vi "Camera.v11.vi"() -> ()   [LabVIEW 2015]
uses:
  Camera Properties.ctl
  Microscope Settings.ctl
  CameraState.ctl
  CameraControlTypeDef.ctl
  ModeEnum.ctl
  Stack Track.ctl
  Stack_State.ctl
  <vilib>/DAQmx/write.llb/DAQmx Write (Digital 1D Wfm NChan NSamp).vi
  <vilib>/DAQmx/write.llb/DAQmx Write (Analog 1D Wfm NChan NSamp).vi
  <vilib>/DAQmx/create/channels.llb/DAQmx Create Channel (AO-Voltage-Basic).vi
  <vilib>/DAQmx/create/channels.llb/DAQmx Create Channel (DO-Digital Output).vi
  <vilib>/Waveform/DWDTOps.llb/DWDT Append Digital Samples.vi
  <vilib>/Waveform/WDTOps.llb/WDT Append Waveforms DBL.vi
  <vilib>/Waveform/WDTOps.llb/WDT Number of Waveform Samples DBL.vi
  <vilib>/DAQmx/configure/timing.llb/DAQmx Timing (Sample Clock).vi
  <vilib>/Waveform/DWDTOps.llb/DWDT Uncompress Digital.vi
  <vilib>/DAQmx/miscellaneous.llb/DAQmx Fill In Error Info.vi
  <vilib>/vision/NI_Vision_Development_Module.lvlib
panel:
  in  "Tab Control":enum32{"Camera Settings", "Recording"}(tab)
  in  "Scans":dbl=1.0 min=0.0 max=10.0 step=0.05
  in  "?":bool
  in  "Microscope Settings":T1={"Mode"=enum."XY", "Slit"={"Scanning Mode"=12.0, "Slit Width /%"=5.0}, "Colour"=[{"Laser"=enum."561", "Filter"=4}], "Exposure/ms"=40.0, "Piezo Position /um"=0.0, "ROI"={"X"={"Start"=0.0, "Step"=1.0, "Range"=2048.0}, "Y"={"Start"=0.0, "Step"=1.0, "Range"=2048.0}, "Z "={"Start"=0.0, "Step"=1.0, "Range"=100.0}}, "Samples per millisecond"=100.0, "Relax/ms"=10.0, "Readout Direction"=2.0, "Trigger Source"=2.0, "Camera Delay /ms"=11.0, "Under Scan"=5.0} {"Under Scan" min=0.0 max=10.0 step=0.05; "ROI"."X"."Range" min=0.0 max=10.0 step=0.05; "ROI"."X"."Step" min=0.0 max=10.0 step=0.05; "ROI"."X"."Start" min=0.0 max=10.0 step=0.05; "ROI"."Y"."Range" min=0.0 max=10.0 step=0.05; "ROI"."Y"."Step" min=0.0 max=10.0 step=0.05; "ROI"."Y"."Start" min=0.0 max=10.0 step=0.05; "ROI"."Z"."Range" min=0.0 max=10.0 step=0.05; "ROI"."Z"."Step" min=0.0 max=10.0 step=0.05; "ROI"."Z"."Start" min=0.0 max=10.0 step=0.05; "Colour"."Filter" items=["Empty"=1, ""=2, ""=3, "561"=4, ""=5, "488"=6]; "Camera Delay /ms" min=0.0 max=10.0 step=0.05; "Trigger Source" items=["Internal"=1.0, "External"=2.0]; "Readout Direction" items=["Forward"=1.0, "Backward"=2.0]; "Slit"."Scanning Mode" items=["Full Frame"=1.0, "Slit Scanning"=12.0]; "Piezo Position /um" min=0.0 max=10.0 step=0.05}
  in  "Scan":bool
  in  "Scan Continuously":bool
  out "error IO":errorcluster
  in  "Advanced DCAM Controls":i32(listbox) caption="Multicolumn Listbox"
  in  "Properties":T2=4211904 items=["SENSOR MODE"=4212128, "CCD MODE"=4212384, "READOUT MODE"=4211872, "ACTIVE VIEW INDEX"=4343136, "BITS PER CHANNEL"=4342976, "IMAGE PIXEL TYPE"=4343296, "BINNING"=4215968, "EXPOSURE TIME"=2049184, "CONTRAST GAIN"=3163312, "CONTRAST OFFSET"=3163328, "LIGHT MODE"=2114720, "SENSITIVITY"=2114992, "PHOTON IMAGING MODE"=2115200, "HIGH DYNAMIC RANGE MODE"=3163360, "WHITE BALANCE"=3163568, "TEMPERATURE"=2115232, "TEMPERATURE TARGET"=2115264, "SENSOR COOLER FAN"=2115296, "LINEBUNDLE HEIGHT"=4212192, "MECHANICAL SHUTTER"=2115488, "BACK FOCUS POSITION"=8422304, "TRIGGER CONNECTOR"=1066432, "TRIGGER SOURCE"=1066144, "OUTPUT TRIGGER SOURCE"=1852576, "TRIGGER GLOBAL EXPOSURE"=2049680, "FIRST TRIGGER BEHAVIOR"=2049696, "CHANNEL SYNC"=1852352, "READOUT DIRECTION"=4211904, "PRE HSYNC COUNT"=1852704, "INTERNAL LINE SPEED"=4191408, "INTERNAL LINE INVERVAL"=4191424]
  out "appended path":path
  in  "Frames":i32
  in  "Imaging Folder":path=path "C:/_DATA/test/a.tif"
  in  "Multicolumn Listbox":i32(listbox)
  out "Image":T3(plugin-control)
  out "Histogram":T4(graph)
  in  "stop":bool
  in  "Record":bool
  in  "Signals Debugger":bool
  in  "Calibration":bool
  in  "MultiD Scan":bool
  in  "Stage Controller":bool
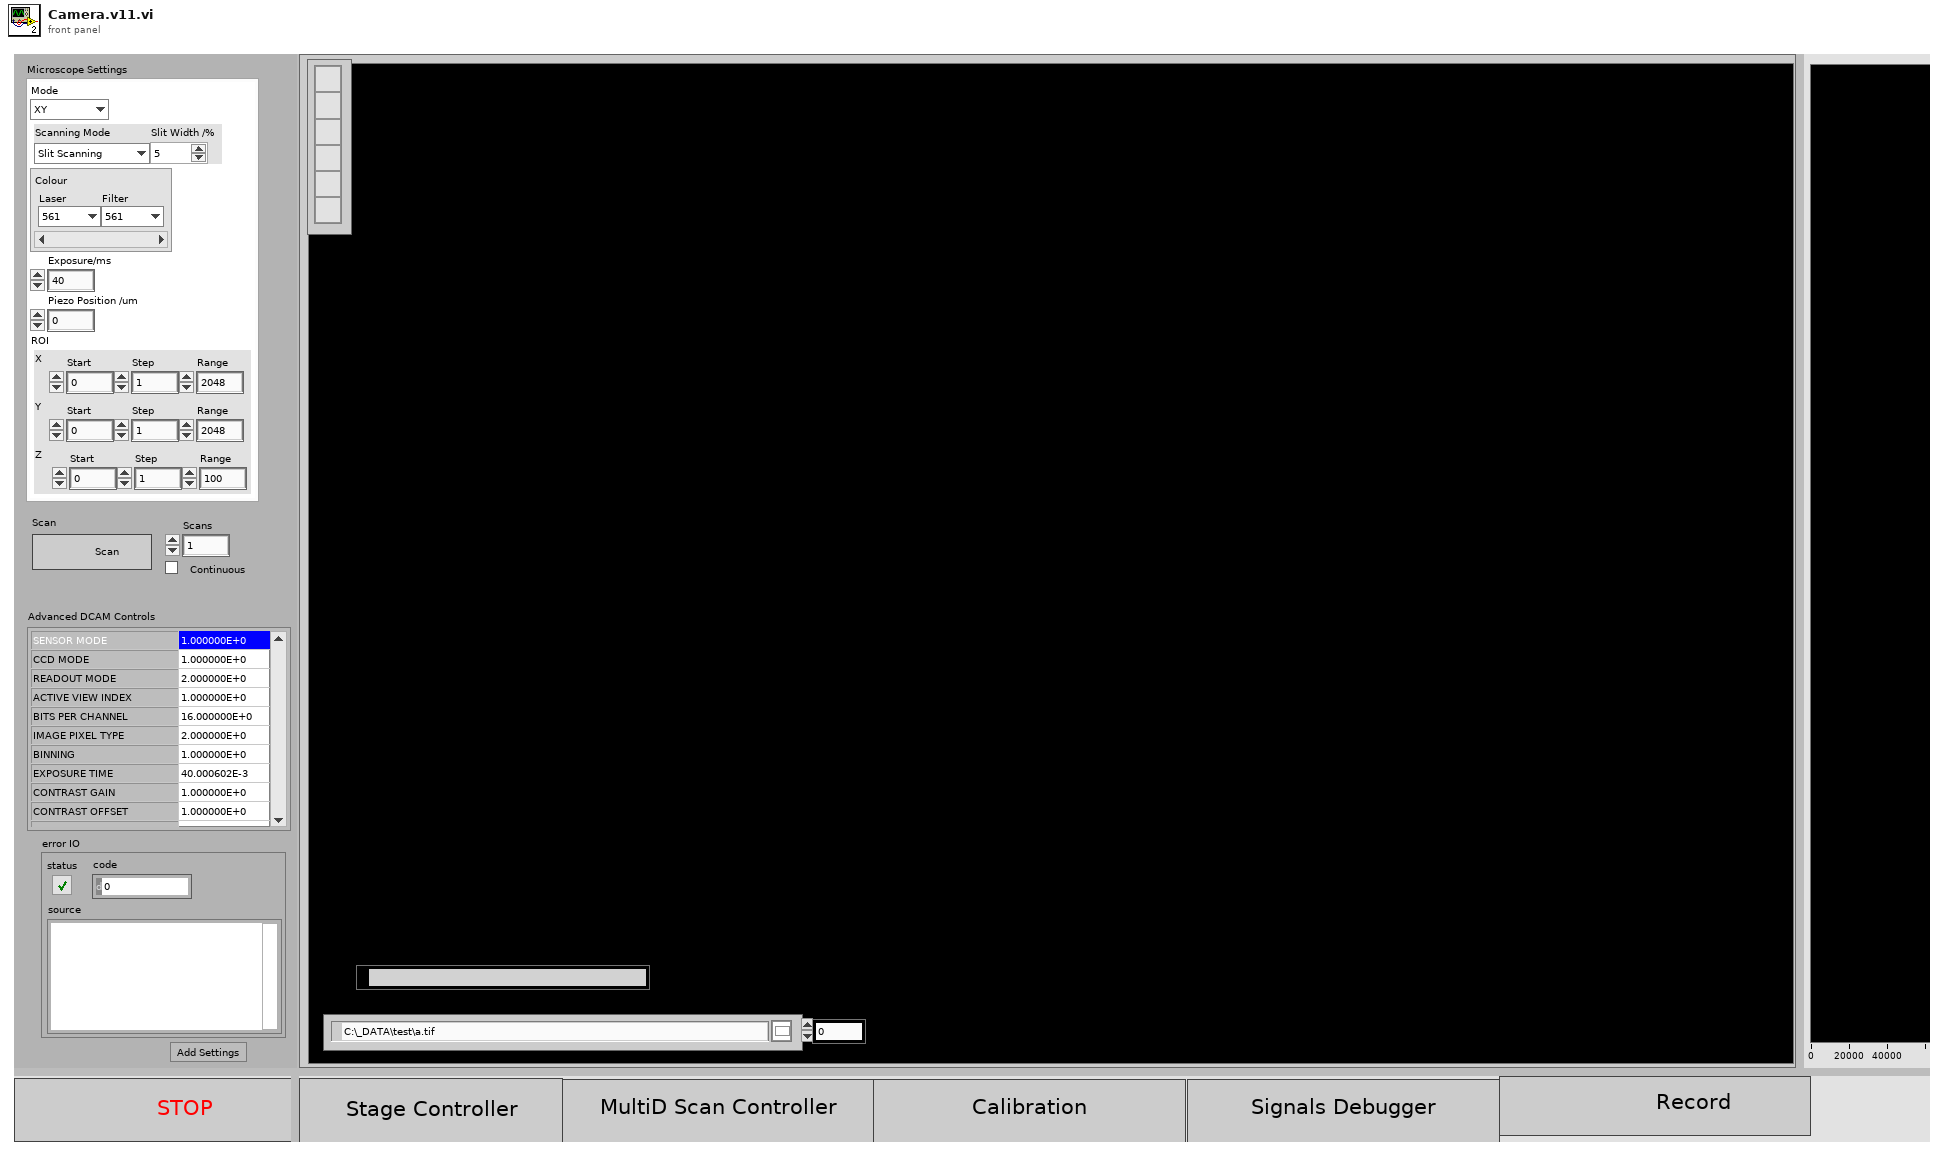
[diagram p1: front panel]
types:
  T1 = typedef "Microscope Settings.ctl" = cluster{"Mode":enum16{"X", "XY", "XYZ", "XYZT", "XYZC"}, "Slit":cluster{"Scanning Mode":dbl, "Slit Width /%":dbl}, "Colour":cluster{"Laser":enum16{"Brightfield", "445", "488", "561", "647"}, "Filter":u16}[], "Exposure/ms":dbl, "Piezo Position /um":dbl, "ROI":cluster{"X":cluster{"Start":dbl, "Step":dbl, "Range":dbl}, "Y":cluster{"Start":dbl, "Step":dbl, "Range":dbl}, "Z ":cluster{"Start":dbl, "Step":dbl, "Range":dbl}}, "Samples per millisecond":dbl, "Relax/ms":dbl, "Readout Direction":dbl, "Trigger Source":dbl, "Camera Delay /ms":dbl, "Under Scan":dbl}
  T2 = typedef "Camera Properties.ctl" = u32
  T3 = typedef "IMAQ Image.ctl" = refnum<image>
  T4 = cluster{"Starting Value":sgl, "Incremental Value":sgl, "Histogram":u32[]}
  T5 = cluster{"height":u32, "width":u32, "datatype":u32}
  T6 = typedef "CameraState.ctl" = enum16{"init", "active", "deinit"}
  T7 = typedef "ModeEnum.ctl" = enum16{"Idle", "generateWaves", "runWaves", "stop"}
  T8 = typedef "CameraControlTypeDef.ctl" = enum16{"Idle", "IntervalLineInt", "Ram Record", "HardDisk Record", "Disengage Update", "Update", "ROI", "Binning", "Scan Mode", "Trigger Mode", "Readout Mode", "Readout Direction", "Preview", "ROIWindow", "Trigger Source"}
  T9 = cluster{"Mode":u32, "Polarity":u32, "Times":u32, "Delay":dbl}
  T10 = typedef "Stack_State.ctl" = cluster{"State":T11, "Stack Number":i32, "Image":u16[][], "Stacks":i32}
  T11 = typedef "Stack Track.ctl" = enum16{"Idle", "Display", "Start Sequence", "Read Disk", "STOP", "Collecting", "End", "Save Image"}
  T12 = enum32{"Invalid", "Standard", "Closed", "Hidden", "Minimized", "Maximized"}
  T13 = typedef "Image Type" = u32
  T14 = cluster{"Analogue Out":waveform(dbl)[], "Digital Out":digitalwaveform[]}
  T15 = cluster{"State":T11, "Timeout":i32, "Data 16":u16[][], "Timeout":i32}
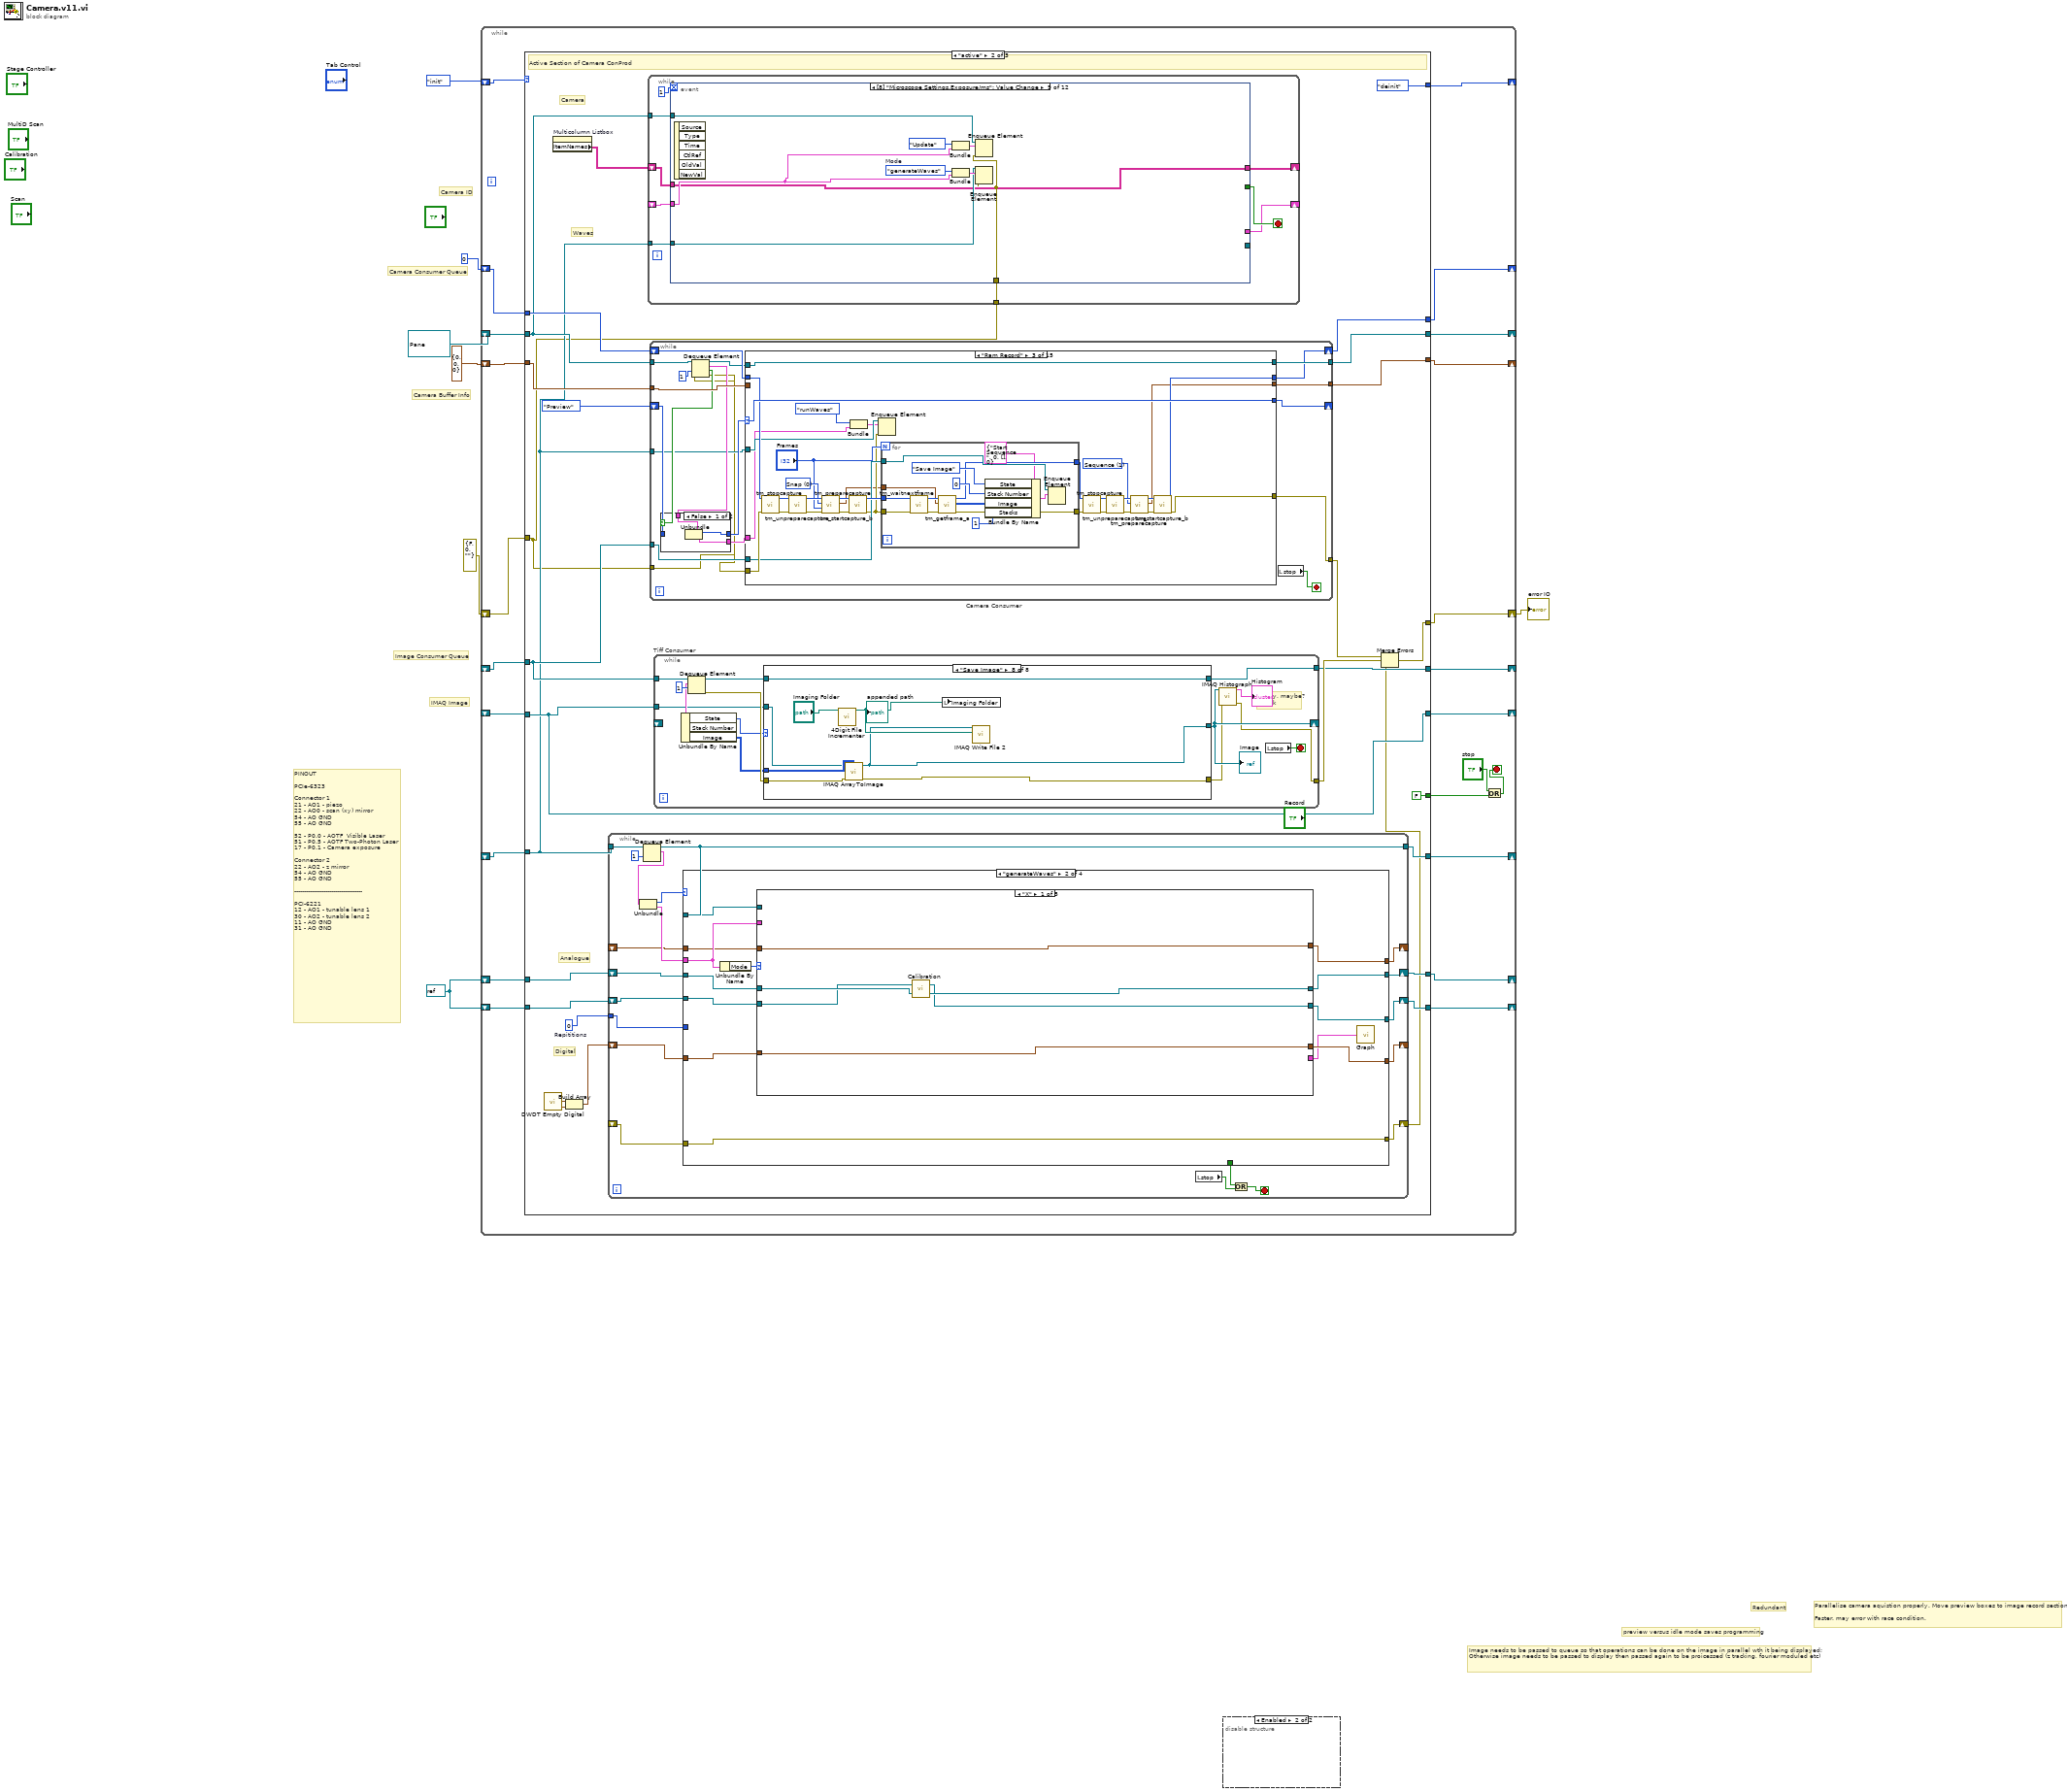
[diagram p0: block diagram]
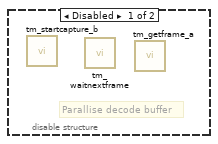
[diagram p2: hidden frame]
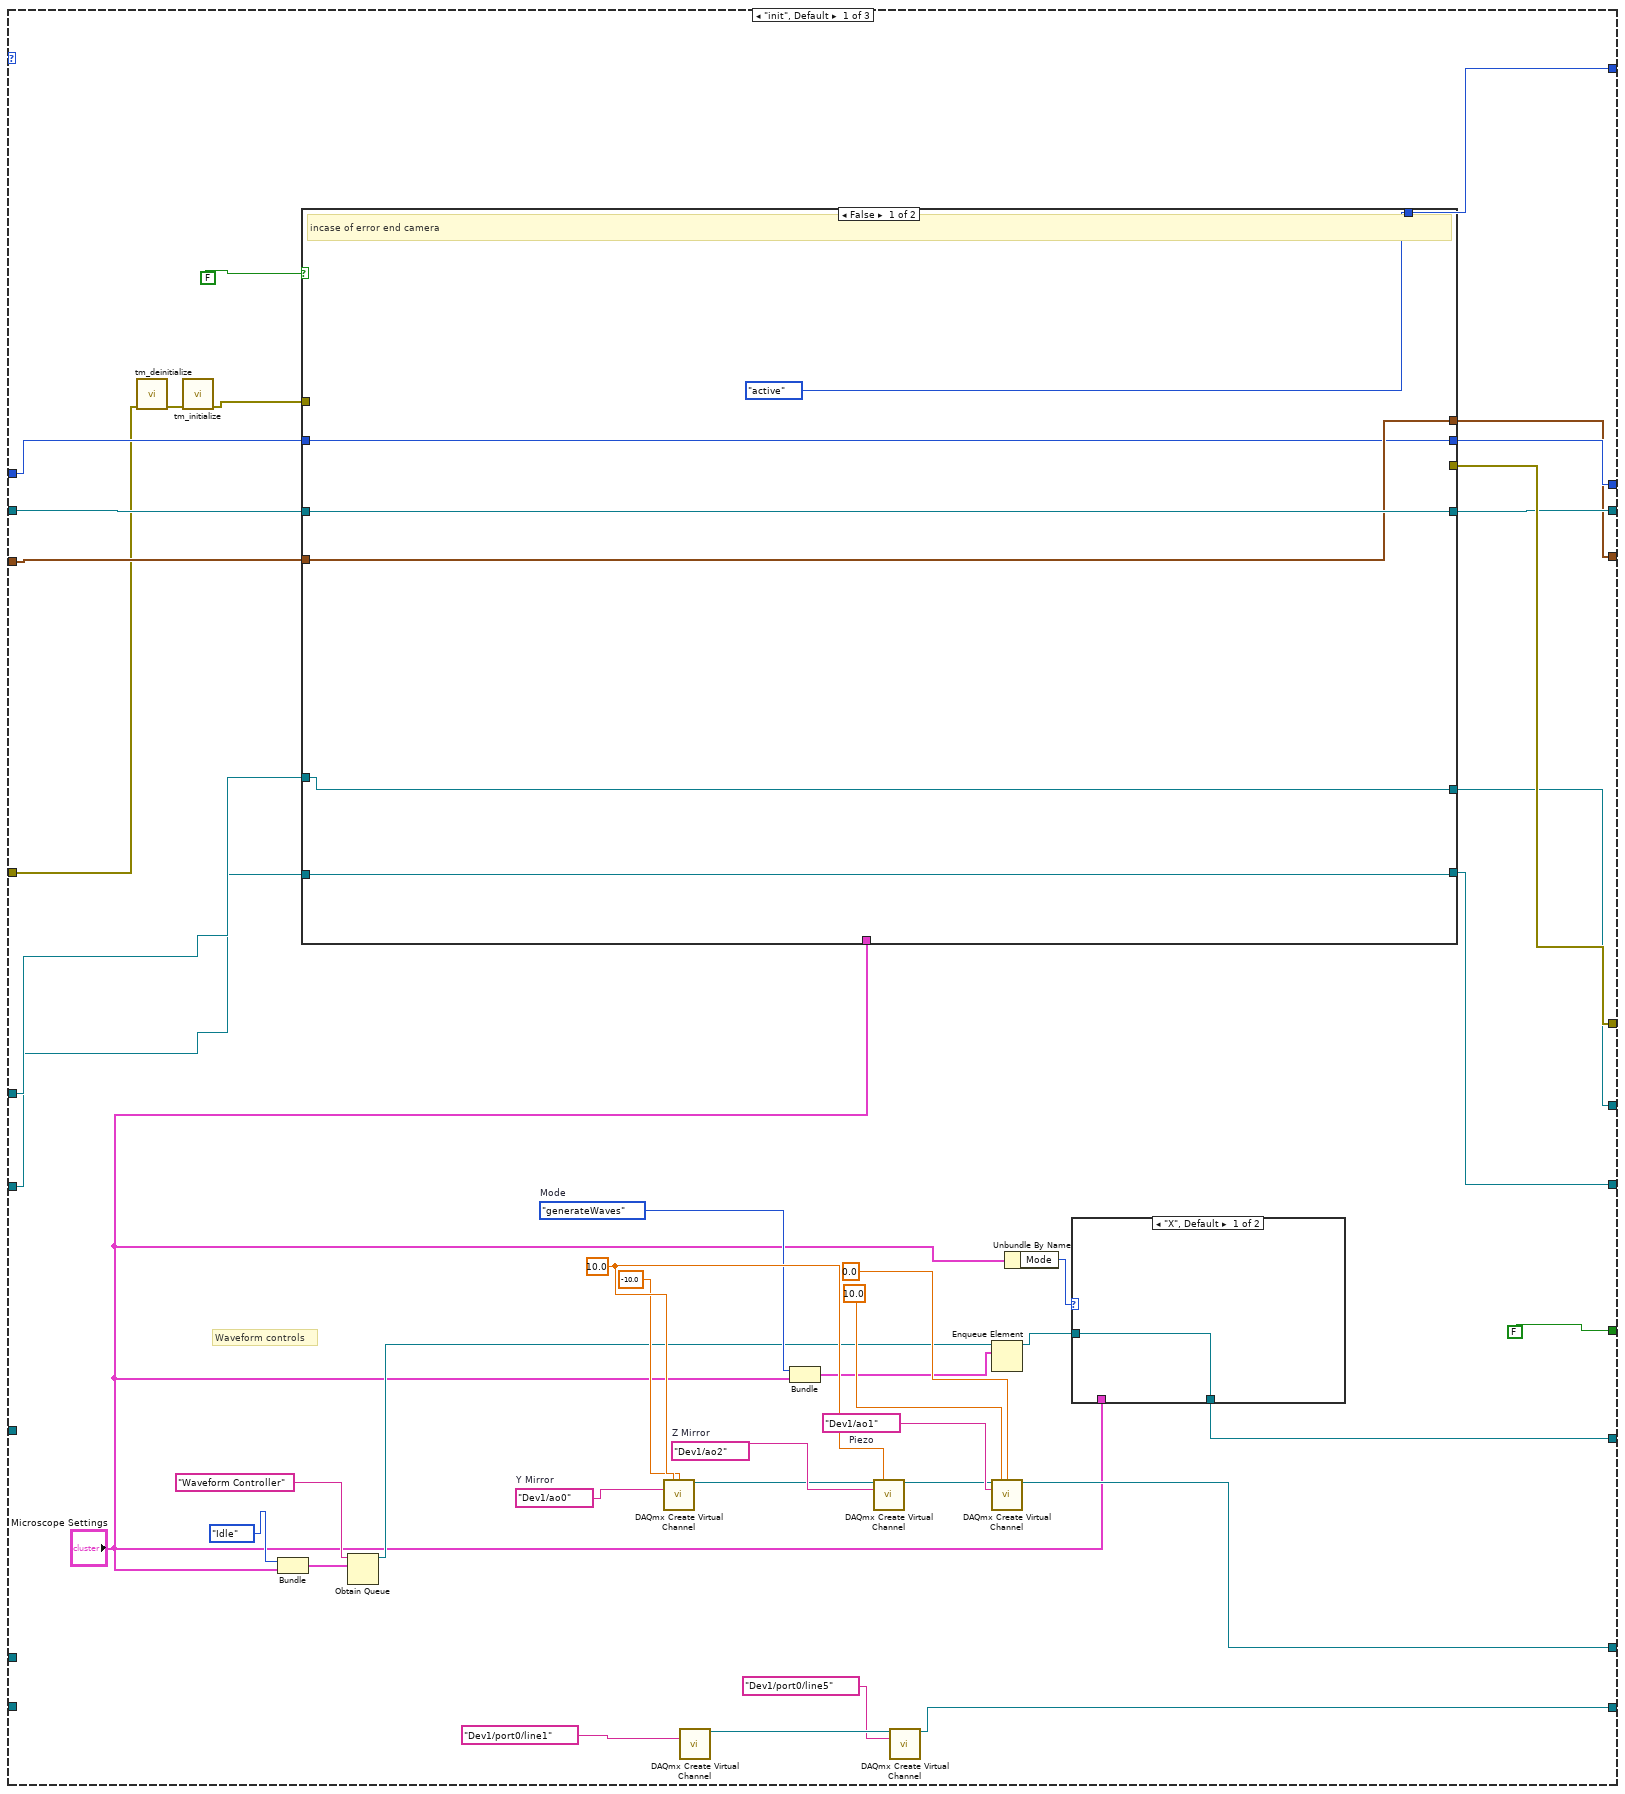
[diagram p3: hidden frame]
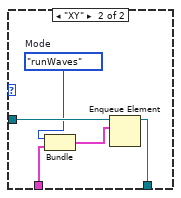
[diagram p4: hidden frame]
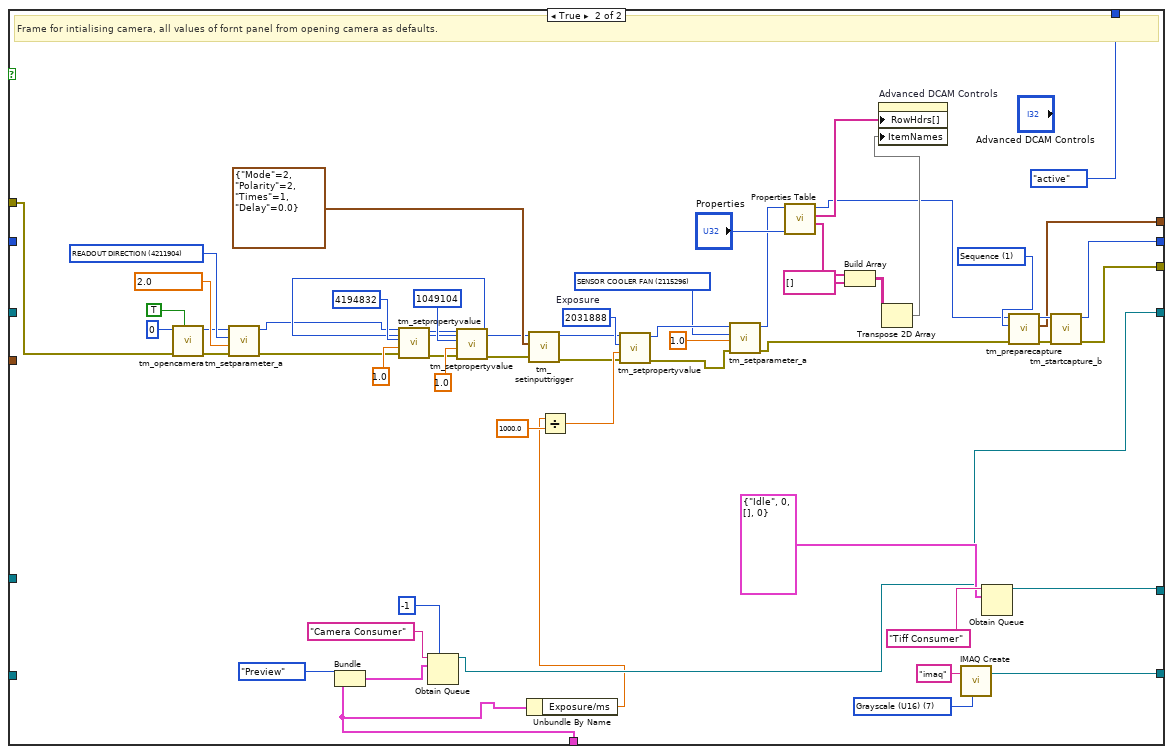
[diagram p5: hidden frame]
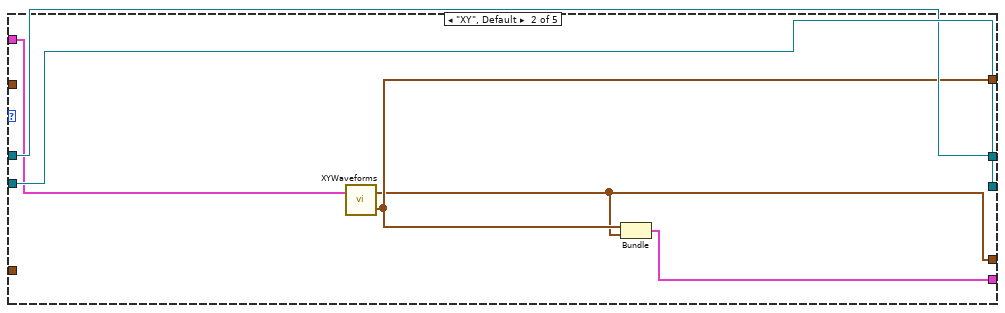
[diagram p7: hidden frame]
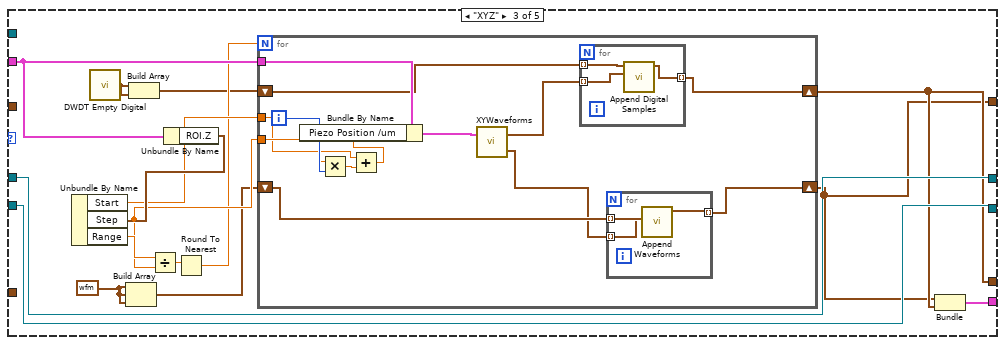
[diagram p8: hidden frame]
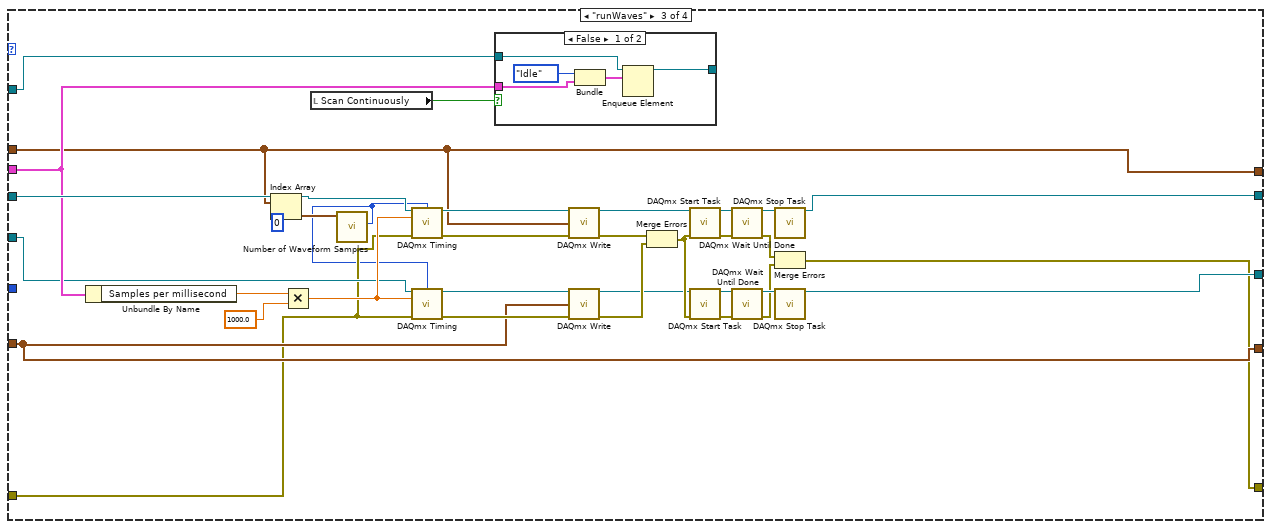
[diagram p11: hidden frame]
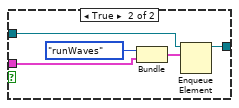
[diagram p12: hidden frame]
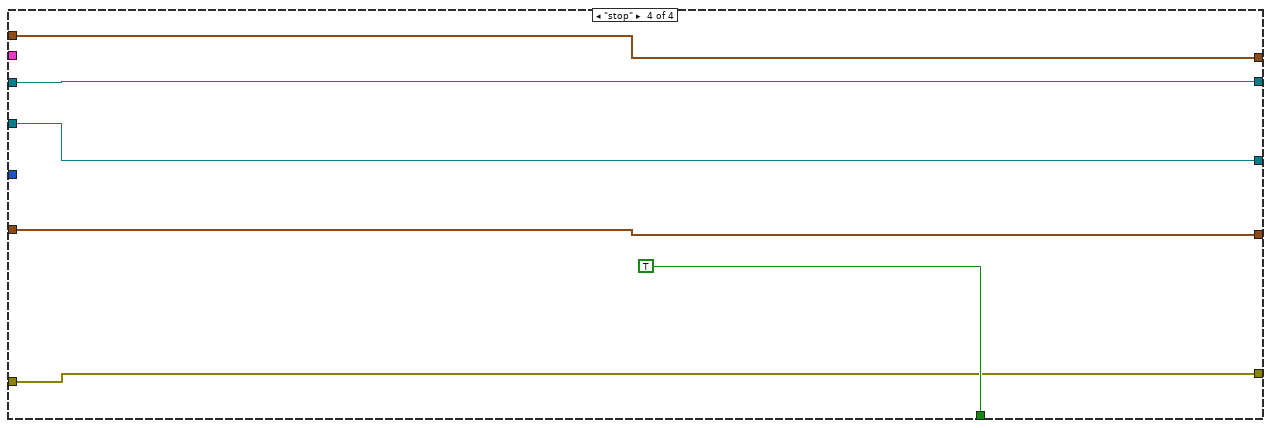
[diagram p13: hidden frame]
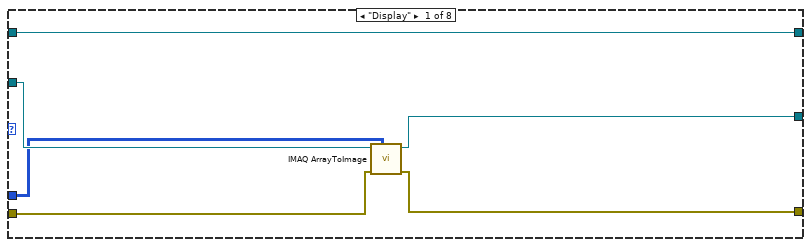
[diagram p14: hidden frame]
diagram:
  w4 = refnum<k21> refnum ("Mirror Z 2")
  # "PINOUT\n\nPCIe-6323\n\nConnector 1\n21 - AO1 - piezo\n22 - AO0 - scan (xy) mirror\n54 - AO GND\n55 - AO GND\n\n52 - P0.0 - AOTF  Visible Laser\n51 - P0.5 - AOTF Two-Photon Laser\n17 - P0.1 - Camera exposure\n\nConnector 2\n22 - AO2 - z mirror\n54 - AO GND\n55 - AO GND\n\n-----------------------------------\n\nPCI-6221\n12 - AO1 - tunable lens 1\n30 - AO2 - tunable lens 2\n11 - AO GND\n31 - AO GND"
  # "IMAQ Image"
  # "Camera Buffer Info"
  # "Image needs to be passed to queue so that operations can be done on the image in parallel wth it being displayed;\nOtherwise image needs to be passed to display then passed again to be proicessed (z tracking, fourier moduled etc)"
  # "preview versus idle mode saves programming"
  # "Parallelise camera aquistion properly. Move preview boxes to image record section.\n\nFaster. may error with race condition."
  # "Redundant"
  # "Image Consumer Queue"
  # "Camera Consumer Queue"
  # "Camera ID"
  n1 = while {
    shift-right: [w30] -> _
    shift-left: CameraState."init" -> [w29]
    shift-right: [w28] -> _
    shift-left: u32 0 ("Handle out") -> [w27]
    shift-right: [w26] -> w6
    shift-left: errorcluster {"status"=FALSE, "code"=0, "source"=""} ("error IO") -> [w25]
    shift-right: [w23] -> _
    shift-left: _ -> [w22]
    shift-right: [w24] -> _
    shift-left: refnum<queue> refnum ("queue out") -> [w21]
    shift-right: [w17] -> _
    shift-left: T5 {"height"=0, "width"=0, "datatype"=0} ("Buffer Info") -> [w16]
    shift-right: [w15] -> _
    shift-left: _ -> [w14]
    shift-right: [w13] -> _
    shift-left: w4 -> [w12]
    shift-right: [w10] -> _
    shift-left: w4 -> [w11]
    shift-right: [w9] -> _
    shift-left: _ -> [w8]
    stop <- w19 stop-if-true
    n2 = case shown="\"active\"" w29 {
      tunnel: [w70 CameraState."deinit" CameraState."init"] -> w30
      tunnel: [w69 w165 w700] -> w28
      tunnel: w27 -> [w48 w166 w700]
      tunnel: [w68 w164 w703] -> w26
      tunnel: w25 -> [w47 w140 w704]
      tunnel: [w67 w161 w687] -> w24
      tunnel: [w66 w160 w683] -> w23
      tunnel: w22 -> [w64 w154 w683]
      tunnel: w21 -> [w65 w152 w687]
      tunnel: [FALSE ("stop") FALSE ("stop") TRUE ("stop")] -> w18
      tunnel: [w62 w157 w697] -> w17
      tunnel: w16 -> [w61 w156 w697]
      tunnel: w14 -> [w59 w153 w696]
      tunnel: [w60 w153 w696] -> w15
      tunnel: w8 -> [_ w141 w682]
      tunnel: [w51 w145 w694] -> w13
      tunnel: w12 -> [_ w148 w694]
      tunnel: w11 -> [_ w147 w692]
      tunnel: [w41 w146 w692] -> w10
      tunnel: [w37 w144 w682] -> w9
      frame "init", Default {
        w45 = ModeEnum."generateWaves"  # Mode
        w54 = tag "Dev1/ao1"  # Piezo
        w55 = tag "Dev1/ao2"  # Z Mirror
        w56 = tag "Dev1/ao0"  # Y Mirror
        w58 = 10.0 ("maximum value")
        # "Waveform controls"
        n3 = call "tm_deinitialize.vi"("error in (no error)"=w47) -> ("error out"=w71:errorcluster)  [unwired: 10 in]
        n4 = call "tm_initialize.vi"("error in (no error)"=w71) -> ("error out"=w31:errorcluster)  [unwired: 7 in, 3 out]
        n5 = Bundle("Mode"=ModeEnum."Idle", "Microscope Settings"="Microscope Settings") -> (w43:cluster{"Mode":T7, "Microscope Settings":T1})  [unwired: 1 in]
        n6 = case shown="False" FALSE {
          tunnel: w31 -> [_ w104]
          tunnel: [CameraState."active" CameraState."active"] -> w70
          tunnel: [_ w135] -> w68
          tunnel: [w79 w133] -> w69
          tunnel: [w82 w123] -> w67
          tunnel: [w81 w130] -> w66
          tunnel: w65 -> [w82 _]
          tunnel: w64 -> [w81 _]
          tunnel: [w80 w128] -> w62
          tunnel: w61 -> [w80 _]
          tunnel: w48 -> [w79 _]
          tunnel: [w78 w125] -> w60
          tunnel: w59 -> [w78 _]
          tunnel: "Microscope Settings" -> [_ w91]
          frame False {
            # "incase of error end camera"
          }
          frame True {
            w101 = u32 2115296 items=["SENSOR MODE"=4212128, "CCD MODE"=4212384, "READOUT MODE"=4211872, "ACTIVE VIEW INDEX"=4343136, "BITS PER CHANNEL"=4342976, "IMAGE PIXEL TYPE"=4343296, "BINNING"=4215968, "EXPOSURE TIME"=2049184, "CONTRAST GAIN"=3163312, "CONTRAST OFFSET"=3163328, "LIGHT MODE"=2114720, "SENSITIVITY"=2114992, "PHOTON IMAGING MODE"=2115200, "HIGH DYNAMIC RANGE MODE"=3163360, "WHITE BALANCE"=3163568, "TEMPERATURE"=2115232, "TEMPERATURE TARGET"=2115264, "SENSOR COOLER FAN"=2115296, "LINEBUNDLE HEIGHT"=4212192, "MECHANICAL SHUTTER"=2115488, "BACK FOCUS POSITION"=8422304, "TRIGGER CONNECTOR"=1066432, "TRIGGER SOURCE"=1066144, "OUTPUT TRIGGER SOURCE"=1852576, "TRIGGER GLOBAL EXPOSURE"=2049680, "FIRST TRIGGER BEHAVIOR"=2049696, "CHANNEL SYNC"=1852352, "READOUT DIRECTION"=4211904, "PRE HSYNC COUNT"=1852704, "INTERNAL LINE SPEED"=4226000, "INTERNAL LINE INTERVAL"=4226016] ("Parameter")
            w110 = u32 2031888  # Exposure
            w121 = sgl 2.0 items=["Forward"=1.0, "Backward"=2.0] ("Readout Direction")
            w122 = u32 4211904 items=["SENSOR MODE"=4212128, "CCD MODE"=4212384, "READOUT MODE"=4211872, "ACTIVE VIEW INDEX"=4343136, "BITS PER CHANNEL"=4342976, "IMAGE PIXEL TYPE"=4343296, "BINNING"=4215968, "EXPOSURE TIME"=2049184, "CONTRAST GAIN"=3163312, "CONTRAST OFFSET"=3163328, "LIGHT MODE"=2114720, "SENSITIVITY"=2114992, "PHOTON IMAGING MODE"=2115200, "HIGH DYNAMIC RANGE MODE"=3163360, "WHITE BALANCE"=3163568, "TEMPERATURE"=2115232, "TEMPERATURE TARGET"=2115264, "SENSOR COOLER FAN"=2115296, "LINEBUNDLE HEIGHT"=4212192, "MECHANICAL SHUTTER"=2115488, "BACK FOCUS POSITION"=8422304, "TRIGGER CONNECTOR"=1066432, "TRIGGER SOURCE"=1066144, "OUTPUT TRIGGER SOURCE"=1852576, "TRIGGER GLOBAL EXPOSURE"=2049680, "FIRST TRIGGER BEHAVIOR"=2049696, "CHANNEL SYNC"=1852352, "READOUT DIRECTION"=4211904, "PRE HSYNC COUNT"=1852704, "INTERNAL LINE SPEED"=4226000, "INTERNAL LINE INTERVAL"=4226016] ("Parameter")
            w127 = T13 7 items=["Grayscale (U8)", "Grayscale (I16)", "Grayscale (SGL)", "Complex (CSG)", "RGB (U32)", "HSL (U32)", "RGB (U64)", "Grayscale (U16)"] ("Image Type")
            w137 = 1 items=["Snap", "Sequence"] ("Capture mode")
            # "Frame for intialising camera, all values of fornt panel from opening camera as defaults."
            n7 = call "tm_opencamera.vi"("Force Open"=TRUE, "error in (no error)"=w104, "Camera Index"=u32 0) -> ("error out"=w119:errorcluster, "Handle out"=w120:u32)  [unwired: 6 in, 1 out]
            n8 = call "tm_setparameter_a.vi"("error in (no error)"=w119, "Value in"=w121, "Parameter"=w122, "Handle in"=w120) -> ("error out"=w89:errorcluster, "Handle out"=w111:u32)  [unwired: 6 in]
            n9 = Bundle("Enum"=CameraControlTypeDef."Preview", "Microscope Settings"=w91) -> (w105:cluster{"Enum":T8, "Microscope Settings":T1})  [unwired: 1 in]
            n10 = call "tm_setpropertyvalue.vi"("error in (no error)"=w89, "Value in"=sgl 1.0, "Property ID"=u32 4194832, "Handle in"=w111) -> ("error out"=w88:errorcluster, "Handle out"=w114:u32)  [unwired: 6 in]
            n11 = Obtain Queue(max queue size (-1, unlimited)=-1, name (unnamed)="Camera Consumer", element data type=w105) -> (queue out=w123:refnum<queue>)  [unwired: 2 in, 2 out]
            n12 = call "tm_setpropertyvalue.vi"("error in (no error)"=w88, "Value in"=sgl 1.0, "Property ID"=u32 1049104, "Handle in"=w114) -> ("error out"=w87:errorcluster, "Handle out"=w112:u32)  [unwired: 6 in]
            n13 = Unbundle By Name(w91) -> ("Exposure/ms"=w90:dbl)
            n14 = call <userlib>:"tm_setinputtrigger.vi"("error in (no error)"=w87, "Parameters"=T9 {"Mode"=2, "Polarity"=2, "Times"=1, "Delay"=0.0}, "Handle in"=w112) -> ("error out"=w86:errorcluster, "Handle out"=w109:u32)  [unwired: 7 in]
            n15 = Divide(x=w90, y=sgl 1000.0) -> (x/y=w107:dbl)
            n16 = call "tm_setpropertyvalue.vi"("error in (no error)"=w86, "Value in"=w107, "Property ID"=w110, "Handle in"=w109) -> ("error out"=w85:errorcluster, "Handle out"=w102:u32)  [unwired: 6 in]
            n17 = call "tm_setparameter_a.vi"("error in (no error)"=w85, "Value in"=1.0, "Parameter"=w101, "Handle in"=w102) -> ("error out"=w84:errorcluster, "Handle out"=w93:u32)  [unwired: 6 in]
            n18 = call "Properties Table.vi"("Properties"="Properties", "Handle In"=w93) -> ("Value Stirngs Out"=w97:string[], "Row Headers"=w98:string[], "Handle Out"=w92:u32)  [unwired: 3 in, 1 out]
            n19 = Build Array(w97, string[] [] ("element")) -> (w95:string[][])
            n20 = Transpose 2D Array(2D array=w95) -> (transposed array=w94:string[][])
            n21 = property on="Advanced DCAM Controls" class="MCListbox (strict)"("RowHdrs[]"=w98, "ItemNames"=w94) -> ()  [unwired: 2 in, 2 out]
            n22 = call "IMAQ Create"("Image Name"="imaq", "Image Type"=w127) -> ("New Image"=w125:T3)  [unwired: 3 in, 1 out]
            n23 = Obtain Queue(name (unnamed)="Tiff Consumer", element data type=T10 {"State"=enum."Idle", "Stack Number"=0, "Image"=[], "Stacks"=0} ("input cluster")) -> (queue out=w130:refnum<queue>)  [unwired: 3 in, 2 out]
            n24 = call "tm_preparecapture.vi"("error in (no error)"=w84, "Capture mode"=w137, "Handle in"=w92) -> ("error out"=w136:errorcluster, "Buffer Info"=w128:T5, "Handle out"=w134:u32)  [unwired: 5 in, 1 out]
            n25 = call "tm_startcapture_b.vi"("error in (no error)"=w136, "Handle in"=w134) -> ("error out"=w135:errorcluster, "Handle out"=w133:u32)  [unwired: 8 in]
          }
        }
        n26 = Obtain Queue(name (unnamed)="Waveform Controller", element data type=w43) -> (queue out=w42:refnum<queue>)  [unwired: 3 in, 2 out]
        n27 = call-poly <vilib>:"DAQmx Create Virtual Channel.vi"("maximum value"=w58, "minimum value"=-10.0, "physical channels"=w56) -> ("task out"=w50:refnum<k21>)  [unwired: 11 in, 1 out]
        n28 = call-poly <vilib>:"DAQmx Create Virtual Channel.vi"("lines"=tag "Dev1/port0/line1") -> ("task out"=w46:refnum<k21>)  [unwired: 13 in, 1 out]
        n29 = Bundle("Mode"=w45, "Microscope Settings"="Microscope Settings") -> (w34:cluster{"Mode":T7, "Microscope Settings":T1})  [unwired: 1 in]
        n30 = call-poly <vilib>:"DAQmx Create Virtual Channel.vi"("task in"=w50, "maximum value"=w58, "physical channels"=w55) -> ("task out"=w49:refnum<k21>)  [unwired: 11 in, 1 out]
        n31 = call-poly <vilib>:"DAQmx Create Virtual Channel.vi"("task in"=w46, "lines"=tag "Dev1/port0/line5") -> ("task out"=w41:refnum<k21>)  [unwired: 12 in, 1 out]
        n32 = Enqueue Element(queue=w42, element=w34) -> (queue out=w38:refnum<queue>)  [unwired: 2 in, 2 out]
        n33 = call-poly <vilib>:"DAQmx Create Virtual Channel.vi"("task in"=w49, "maximum value"=10.0 ("minimum value"), "minimum value"=0.0 ("maximum value"), "physical channels"=w54) -> ("task out"=w51:refnum<k21>)  [unwired: 10 in, 1 out]
        n34 = Unbundle By Name("Microscope Settings") -> ("Mode"=w33:enum16{"X", "XY", "XYZ", "XYZT", "XYZC"})
        n35 = case shown="\"X\", Default" w33 {
          tunnel: w38 -> [w72 w77]
          tunnel: [w72 w75] -> w37
          tunnel: "Microscope Settings" -> [_ w74]
          frame "X", Default {
          }
          frame "XY" {
            w73 = ModeEnum."runWaves"  # Mode
            n36 = Bundle("Mode"=w73, "Microscope Settings"=w74) -> (w76:cluster{"Mode":T7, "Microscope Settings":T1})  [unwired: 1 in]
            n37 = Enqueue Element(queue=w77, element=w76) -> (queue out=w75:refnum<queue>)  [unwired: 2 in, 2 out]
          }
        }
      }
      frame "active" {
        w151 = 0  # Repititions
        # "Waves"
        # "Camera"
        # "Digital"
        # "Analogue"
        # "Active Section of Camera ConProd"
        n38 = call <vilib>:"DWDT Empty Digital.vi"() -> ("digital waveform out"=w149:digitalwaveform)  [unwired: 5 in]
        n39 = property on="Multicolumn Listbox" class="MCListbox (strict)"() -> ("ItemNames"=w142:string[][])  [unwired: 2 in, 2 out]
        n40 = Build Array(w149, w149) -> (w150:digitalwaveform[])
        n41 = while {
          tunnel: w141 -> [w186]
          shift-right: [w182] -> _
          shift-left: _ -> [w181]
          tunnel: w151 -> [w180]
          shift-right: [w176] -> w145
          shift-left: w148 -> [w175]
          shift-right: [w179] -> _
          shift-left: w150 -> [w178]
          shift-right: [w174] -> w146
          shift-left: w147 -> [w173]
          tunnel: [w172] -> w144
          shift-right: [w171] -> w143
          shift-left: _ -> [w170]
          stop <- w167 stop-if-true
          n42 = Dequeue Element(queue=w186, timeout in ms (-1)=1) -> (queue out=w172:refnum<queue>, element=w185:cluster{"Mode":T7, "Microscope Settings":T1})  [unwired: 1 in, 2 out]
          n43 = Unbundle(w185) -> ("Mode"=w184:T7, "Microscope Settings"=w183:T1)
          n44 = case shown="\"generateWaves\"" w184 {
            tunnel: [_ _ _ TRUE] -> w169
            tunnel: w183 -> [_ w203 w288 _]
            tunnel: [w191 w204 w287 w309] -> w182
            tunnel: w181 -> [w191 w195 w287 w309]
            tunnel: w180 -> [_ _ _ _]
            tunnel: w172 -> [_ w194 w289 _]
            tunnel: [w188 w199 w267 w308] -> w174
            tunnel: [w189 w197 w282 w307] -> w176
            tunnel: w175 -> [w189 w196 w290 w307]
            tunnel: [w190 w202 w269 w306] -> w179
            tunnel: w178 -> [w190 w201 w269 w306]
            tunnel: w173 -> [w188 w200 w278 w308]
            tunnel: [w187 w193 w264 w304] -> w171
            tunnel: w170 -> [w187 w193 w263 w304]
            frame "Idle", Default {
            }
            frame "generateWaves" {
              n45 = Unbundle By Name(w203) -> ("Mode"=w198:enum16{"X", "XY", "XYZ", "XYZT", "XYZC"})
              n46 = case shown="\"X\"" w198 {
                tunnel: [w210 w213 w221 w255 w259] -> w204
                tunnel: w203 -> [_ w214 w232 _ _]
                tunnel: [w209 w212 w225 w252 w256] -> w202
                tunnel: w201 -> [w209 _ _ w252 w256]
                tunnel: w200 -> [w206 w216 w226 w253 w257]
                tunnel: [w205 w216 w226 w253 w257] -> w199
                tunnel: [w208 w215 w227 w254 w258] -> w197
                tunnel: w196 -> [w207 w215 w227 w254 w258]
                tunnel: w195 -> [w210 _ _ w255 w259]
                tunnel: w194 -> [_ _ _ _ _]
                tunnel: [_ w211 w222 _ _] -> w192
                frame "X" {
                  n47 = call "Calibration.vi"("Analogue In"=w207, "Digital In"=w206) -> ("Analogue In Out"=w208:refnum<k21>, "Digital Out"=w205:refnum<k21>)
                }
                frame "XY", Default {
                  n48 = call "XYWaveforms.vi"("Microscope Settings"=w214) -> ("Analogue Out"=w213:waveform(dbl)[], "Digital Out"=w212:digitalwaveform[])  [unwired: 1 in]
                  n49 = Bundle("Analogue Out"=w213, "Digital Out"=w212) -> (w211:T14)  [unwired: 1 in]
                }
                frame "XYZ" {
                  w217 = waveform(dbl) {"t0"=timestamp(0 s since 1904-01-01), "dt"=1.0, "Y"=[]} ("Waveform")
                  n50 = call <vilib>:"DWDT Empty Digital.vi"() -> ("digital waveform out"=w220:digitalwaveform)  [unwired: 5 in]
                  n51 = Build Array(w217, w217, w217) -> (w218:waveform(dbl)[])
                  n52 = Build Array(w220, w220) -> (w219:digitalwaveform[])
                  n53 = Unbundle By Name(w232) -> ("ROI.Z"=w231:cluster{"Start":dbl, "Step":dbl, "Range":dbl})
                  n54 = Unbundle By Name(w231) -> ("Start"=w230:dbl, "Step"=w228:dbl, "Range"=w229:dbl)
                  n55 = Divide(x=w229, y=w228) -> (x/y=w224:dbl)
                  n56 = Round To Nearest(number=w224) -> (nearest integer value=w223:dbl)
                  n57 = for {
                    N: w223 -> [_]
                    tunnel: w232 -> [w245]
                    tunnel: w228 -> [w241]
                    tunnel: w230 -> [w240]
                    shift-right: [w236] -> w221
                    shift-left: w218 -> [w238]
                    shift-right: [w234] -> w225
                    shift-left: w219 -> [w233]
                    i -> [w242]
                    n58 = Multiply(x=w241, y=w242) -> (x*y=w243:dbl)
                    n59 = Add(x=w240, y=w243) -> (x+y=w239:dbl)
                    n60 = Bundle By Name(cluster=w245, "Piezo Position /um"=w239) -> (w244:T1)
                    n61 = call "XYWaveforms.vi"("Microscope Settings"=w244) -> ("Analogue Out"=w237:waveform(dbl)[], "Digital Out"=w235:digitalwaveform[])  [unwired: 1 in]
                    n62 = for {
                      tunnel: w235 -> [w247] mode=indexing
                      tunnel: w233 -> [w248] mode=indexing
                      tunnel: [w246] -> w234 mode=indexing
                      n63 = call-poly <vilib>:"Append Digital Samples.vi"("digital waveform B"=w247, "digital waveform A"=w248) -> ("digital waveform out"=w246:digitalwaveform)  [unwired: 8 in, 1 out]
                    }
                    n64 = for {
                      tunnel: w237 -> [w250] mode=indexing
                      tunnel: w238 -> [w251] mode=indexing
                      tunnel: [w249] -> w236 mode=indexing
                      n65 = call-poly <vilib>:"Append Waveforms.vi"("waveform B"=w250, "waveform A"=w251) -> ("waveform out"=w249:waveform(dbl))  [unwired: 8 in, 1 out]
                    }
                  }
                  n66 = Bundle(w221, w225) -> (w222:cluster{waveform(dbl)[], digitalwaveform[]})  [unwired: 1 in]
                }
                frame "XYZT" {
                }
                frame "XYZC" {
                }
              }
              n67 = call "Graph.vi"("Cluster"=w192) -> ()
            }
            frame "runWaves" {
              n68 = Unbundle By Name(w288) -> ("Samples per millisecond"=w260:dbl)
              n69 = Index Array(array=w287, index=0) -> (element=w285:waveform(dbl))
              n70 = Multiply(x=w260, y=1000.0) -> (x*y=w280:dbl)
              n71 = local read "Scan Continuously"() -> (w281:bool)
              n72 = call-poly <vilib>:"Number of Waveform Samples.vi"("waveform in"=w285) -> ("number of samples"=w261:i32)  [unwired: 8 in, 2 out]
              n73 = call-poly <vilib>:"DAQmx Timing.vi"("task/channels in"=w290, "samples per channel"=w261, "rate"=w280, "error in"=w263) -> ("task out"=w293:refnum<k21>, "error out"=w284:errorcluster)  [unwired: 10 in]
              n74 = call-poly <vilib>:"DAQmx Timing.vi"("task/channels in"=w278, "samples per channel"=w261, "rate"=w280, "error in"=w263) -> ("task out"=w279:refnum<k21>, "error out"=w276:errorcluster)  [unwired: 10 in]
              n75 = case shown="False" w281 {
                tunnel: w289 -> [w295 w303]
                tunnel: [w296 w302] -> _
                tunnel: w288 -> [w297 w301]
                frame False {
                  n76 = Bundle("Mode"=ModeEnum."Idle", "Microscope Settings"=w297) -> (w298:cluster{"Mode":T7, "Microscope Settings":T1})  [unwired: 1 in]
                  n77 = Enqueue Element(queue=w295, element=w298) -> (queue out=w296:refnum<queue>)  [unwired: 2 in, 2 out]
                }
                frame True {
                  n78 = Bundle("Mode"=ModeEnum."runWaves", "Microscope Settings"=w301) -> (w300:cluster{"Mode":T7, "Microscope Settings":T1})  [unwired: 1 in]
                  n79 = Enqueue Element(queue=w303, element=w300) -> (queue out=w302:refnum<queue>)  [unwired: 2 in, 2 out]
                }
              }
              n80 = call-poly <vilib>:"DAQmx Write.vi"("task/channels in"=w293, "data"=w287, "error in"=w284) -> ("task out"=w271:refnum<k21>, "error out"=w274:errorcluster)  [unwired: 10 in, 1 out]
              n81 = call-poly <vilib>:"DAQmx Write.vi"("task/channels in"=w279, "data"=w269, "error in"=w276) -> ("task out"=w270:refnum<k21>, "error out"=w273:errorcluster)  [unwired: 10 in, 1 out]
              n82 = Merge Errors(w274, w273) -> (w272:errorcluster)
              n83 = call <vilib>:"DAQmx Start Task.vi"("task/channels in"=w271, "error in"=w272) -> ("task out"=w292:refnum<k21>, "error out"=w291:errorcluster)  [unwired: 12 in]
              n84 = call <vilib>:"DAQmx Start Task.vi"("task/channels in"=w270, "error in"=w272) -> ("task out"=w277:refnum<k21>, "error out"=w275:errorcluster)  [unwired: 12 in]
              n85 = call <vilib>:"DAQmx Wait Until Done.vi"("task/channels in"=w292, "error in"=w291) -> ("task out"=w283:refnum<k21>, "error out"=w266:errorcluster)  [unwired: 12 in]
              n86 = call <vilib>:"DAQmx Wait Until Done.vi"("task/channels in"=w277, "error in"=w275) -> ("task out"=w268:refnum<k21>, "error out"=w265:errorcluster)  [unwired: 12 in]
              n87 = call <vilib>:"DAQmx Stop Task.vi"("task/channels in"=w283) -> ("task out"=w282:refnum<k21>)  [unwired: 13 in, 1 out]
              n88 = Merge Errors(w266, w265) -> (w264:errorcluster)
              n89 = call <vilib>:"DAQmx Stop Task.vi"("task/channels in"=w268) -> ("task out"=w267:refnum<k21>)  [unwired: 13 in, 1 out]
            }
            frame "stop" {
            }
          }
          n90 = local read "stop"() -> (w168:bool)
          n91 = Or(x=w169, y=w168) -> (x .or. y?=w167:bool)
        }
        n92 = while {
          tunnel: w152 -> [w594]
          shift-right: [w593] -> _
          shift-left: _ -> [w592]
          tunnel: w141 -> [w590]
          shift-right: [w589] -> _
          shift-left: w142 -> [w588]
          tunnel: w140 -> [w587]
          stop <- w595 stop-if-true
          n93 = event shown="[8] \"Microscope Settings.Exposure/ms\": Value Change" {
            selector: _ -> [_ _ _ _ _ _ _ _ _ _ _ _]
            dyn-events: _ -> [_ _ _ _ _ _ _ _ _ _ _ _]
            timeout: 1 -> [_ _ _ _ _ _ _ _ _ _ _ _]
            tunnel: [w604 _ _ _ _ _ _ _ _ _ _ _] -> w595
            tunnel: w594 -> [w599 _ w618 w623 w630 _ w640 _ w654 _ _ _]
            tunnel: [w597 _ w612 w621 _ _ _ _ _ _ _ w681] -> w593
            tunnel: w592 -> [w597 w610 w612 w621 w626 w633 w639 w648 w655 _ w669 _]
            tunnel: [_ _ _ w622 _ _ _ _ _ _ w668 _] -> _
            tunnel: w590 -> [w598 _ w617 w622 w627 w634 _ w647 w653 _ w667 _]
            tunnel: [w596 w605 w611 w619 w629 w637 w641 w646 w652 w661 w665 w680] -> w589
            tunnel: w588 -> [w596 w607 w611 w619 w629 w637 w641 w646 w652 w661 w665 w680]
            tunnel: w587 -> [_ _ _ _ _ _ _ _ w651 _ _ _]
            event "stop": Value Change {
              w602 = ModeEnum."stop"  # Mode
              n94 = event-data() -> ()  [unwired: 1 in, 6 out]
              n95 = Bundle("Enum"=CameraControlTypeDef."Idle", "Value"=w597) -> (w600:cluster{"Enum":T8, "Value":T1})  [unwired: 1 in]
              n96 = Bundle("Mode"=w602, "Value"=w597) -> (w601:cluster{"Mode":T7, "Value":T1})  [unwired: 1 in]
              n97 = Enqueue Element(queue=w599, element=w600) -> ()  [unwired: 2 in, 3 out]
              n98 = Enqueue Element(queue=w598, element=w601) -> ()  [unwired: 2 in, 3 out]
              n99 = local read "stop"() -> (w604:bool)
            }
            event Value Change {
              n100 = event-data() -> ()  [unwired: 1 in, 6 out]
              n101 = Flatten To XML(anything=w610) -> (xml string=w609:string)
              n102 = Build Array("Experiment 1" ("element"), w609) -> (w606:string[])
              n103 = Build Array (concatenate)(w607, w606) -> (w605:string[][])
              n104 = property on="Multicolumn Listbox" class="MCListbox (strict)"("ItemNames"=w605) -> ()  [unwired: 2 in, 2 out]
            }
            event Value Change {
              w615 = ModeEnum."generateWaves"  # Mode
              # "Live video for Calibration and 2D\nScan Modes.\n\nIdle Video for MultiD Scan modes\nUNTIL Begin Scan Button pressed?\n\nMultiD is waiting for trigger"
              n105 = event-data() -> ()  [unwired: 1 in, 6 out]
              n106 = Bundle("Enum"=CameraControlTypeDef."Trigger Source", "Value"=w612) -> (w613:cluster{"Enum":T8, "Value":T1})  [unwired: 1 in]
              n107 = Bundle("Mode"=w615, "Value"=w612) -> (w614:cluster{"Mode":T7, "Value":T1})  [unwired: 1 in]
              n108 = Enqueue Element(queue=w618, element=w613) -> ()  [unwired: 2 in, 3 out]
              n109 = Enqueue Element(queue=w617, element=w614) -> ()  [unwired: 2 in, 3 out]
            }
            event Value Change {
              n110 = event-data() -> ()  [unwired: 1 in, 6 out]
              n111 = Bundle("Enum"=CameraControlTypeDef."Readout Mode", "Value"=w621) -> (w620:cluster{"Enum":T8, "Value":T1})  [unwired: 1 in]
              n112 = Enqueue Element(queue=w623, element=w620) -> ()  [unwired: 2 in, 3 out]
            }
            event Value Change {
              w625 = ModeEnum."generateWaves"  # Mode
              n113 = event-data() -> ()  [unwired: 1 in, 6 out]
              n114 = Bundle("Enum"=CameraControlTypeDef."ROI", "Value"=w626) -> (w631:cluster{"Enum":T8, "Value":T1})  [unwired: 1 in]
              n115 = Bundle("Mode"=w625, "Value"=w626) -> (w628:cluster{"Mode":T7, "Value":T1})  [unwired: 1 in]
              n116 = Enqueue Element(queue=w630, element=w631) -> ()  [unwired: 2 in, 3 out]
              n117 = Enqueue Element(queue=w627, element=w628) -> ()  [unwired: 2 in, 3 out]
            }
            event Value Change {
              w635 = ModeEnum."generateWaves"  # Mode
              n118 = event-data() -> ()  [unwired: 1 in, 6 out]
              n119 = Bundle("Mode"=w635, "Value"=w633) -> (w636:cluster{"Mode":T7, "Value":T1})  [unwired: 1 in]
              n120 = Enqueue Element(queue=w634, element=w636) -> ()  [unwired: 2 in, 3 out]
            }
            event "Record": Value Change {
              n121 = event-data() -> ("NewVal"=w638:bool)  [unwired: 1 in, 5 out]
              n122 = case shown="True" w638 {
                tunnel: w640 -> [_ w645]
                tunnel: w639 -> [_ w643]
                frame False {
                }
                frame True {
                  n123 = Bundle("Enum"=CameraControlTypeDef."Ram Record", "Value"=w643) -> (w642:cluster{"Enum":T8, "Value":T1})  [unwired: 1 in]
                  n124 = Enqueue Element(queue=w645, element=w642) -> ()  [unwired: 2 in, 3 out]
                }
              }
            }
            event Value Change {
              w650 = ModeEnum."generateWaves"  # Mode
              n125 = event-data() -> ()  [unwired: 1 in, 6 out]
              n126 = Bundle("Mode"=w650, "Value"=w648) -> (w649:cluster{"Mode":T7, "Value":T1})  [unwired: 1 in]
              n127 = Enqueue Element(queue=w647, element=w649) -> ()  [unwired: 2 in, 3 out]
            }
            event Value Change {
              w658 = ModeEnum."generateWaves"  # Mode
              n128 = event-data() -> ()  [unwired: 1 in, 6 out]
              n129 = Bundle("Enum"=CameraControlTypeDef."Update", "Value"=w655) -> (w656:cluster{"Enum":T8, "Value":T1})  [unwired: 1 in]
              n130 = Bundle("Mode"=w658, "Value"=w655) -> (w657:cluster{"Mode":T7, "Value":T1})  [unwired: 1 in]
              n131 = Enqueue Element(queue=w654, element=w656, error in (no error)=w651) -> ()  [unwired: 1 in, 3 out]
              n132 = Enqueue Element(queue=w653, element=w657, error in (no error)=w651) -> ()  [unwired: 1 in, 3 out]
            }
            event "Signals Debugger": Value Change {
              n133 = event-data() -> ()  [unwired: 1 in, 6 out]
              n134 = case shown="True" "Signals Debugger" {
                frame False {
                }
                frame True {
                  n135 = vi-ref "Graph.vi"() -> (w662:refnum<vi>)
                  n136 = invoke class="VI" method="FP.Open"(reference=w662, "Activate"=TRUE ("Front Panel Window:Open"), "State"=T12."Standard") -> ()  [unwired: 2 in, 5 out]
                }
              }
            }
            event "Scan": Value Change {
              n137 = event-data() -> ("NewVal"=w666:bool)  [unwired: 1 in, 5 out]
              n138 = case shown="True" w666 {
                tunnel: w669 -> [_ w674]
                tunnel: [w670 w673] -> w668
                tunnel: w667 -> [w670 w672]
                frame False {
                }
                frame True {
                  n139 = for {
                    N: "Scans" -> [_]
                    tunnel: w674 -> [w676]
                    tunnel: [w675] -> w673
                    tunnel: w672 -> [w679]
                    w678 = ModeEnum."runWaves"  # Mode
                    n140 = Bundle("Mode"=w678, "Value"=w676) -> (w677:cluster{"Mode":T7, "Value":T1})  [unwired: 1 in]
                    n141 = Enqueue Element(queue=w679, element=w677) -> (queue out=w675:refnum<queue>)  [unwired: 2 in, 2 out]
                  }
                }
              }
            }
            event Timeout {
              n142 = event-data() -> ()  [unwired: 1 in, 3 out]
              n143 = property on="Microscope Settings" class="Clust (strict)"() -> ("Value"=w681:T1)  [unwired: 2 in, 2 out]
            }
          }
        }
        n144 = while "Camera Consumer" {
          tunnel: w140 -> [w356]
          tunnel: [w360] -> w162
          tunnel: w152 -> [w368]
          tunnel: [w375] -> w161
          shift-right: [w374] -> _
          shift-left: CameraControlTypeDef."Preview" ("Enum") -> [w364]
          tunnel: [w371] -> w157
          tunnel: w156 -> [w370]
          tunnel: w154 -> [w363]
          shift-right: [w372] -> w165
          shift-left: w166 -> [w373]
          tunnel: w141 -> [w358]
          stop <- w359 stop-if-true
          n145 = Dequeue Element(queue=w368, timeout in ms (-1)=1, error in (no error)=w356) -> (queue out=w367:refnum<queue>, element=w362:cluster{"Enum":T8, "Microscope Settings":T1}, timed out?=w366:bool, error out=w357:errorcluster)
          n146 = case shown="False" w366 {
            tunnel: [w377 CameraControlTypeDef."Preview" ("Enum")] -> w365
            tunnel: w364 -> [_ _]
            tunnel: w362 -> [w378 _]
            tunnel: [w376 _] -> w361
            frame False {
              n147 = Unbundle(w378) -> ("Enum"=w377:T8, "Microscope Settings"=w376:T1)
            }
            frame True {
            }
          }
          n148 = case shown="\"Ram Record\"" w365 {
            selector: w365 -> [w383 w388 w420 w439 w444 w455 w460 w465 w470 w475 w508 w526 _ w555 _]
            tunnel: w367 -> [w382 w389 w421 w440 w445 w456 w461 w466 w471 w476 _ w522 w537 w557 w576]
            tunnel: [w382 w389 w421 w440 w445 w456 w461 w466 w471 w476 _ w522 w537 w557 w576] -> w375
            tunnel: w357 -> [w384 w387 w417 w438 w443 w454 w459 w464 w469 w474 w503 w525 w529 w554 w567]
            tunnel: [w384 w387 w399 w438 w443 w454 w459 w464 w469 w474 w477 w525 w528 w554 w568] -> w360
            tunnel: [w383 w388 w420 w439 w444 w455 w460 w465 w470 w475 w508 w526 CameraControlTypeDef."Preview" ("Enum") w555 w558] -> w374
            tunnel: w373 -> [w381 w386 w401 w437 w441 w452 w458 w463 w468 w473 w505 w524 w535 w556 w570]
            tunnel: [w381 w386 w400 w437 w441 w451 w458 w463 w468 w473 w479 w524 w533 w556 w569] -> w372
            tunnel: [w380 w385 w390 w436 w442 w453 w457 w462 w467 w472 w507 w523 w531 w553 w571] -> w371
            tunnel: w370 -> [w380 w385 _ w436 w442 w453 w457 w462 w467 w472 w507 w523 w531 w553 _]
            tunnel: w363 -> [_ _ w410 _ _ _ _ _ _ _ _ _ w530 _ _]
            tunnel: w361 -> [_ _ w395 _ _ w450 _ _ _ _ w502 _ _ _ w560]
            tunnel: w358 -> [_ _ w397 _ _ _ _ _ _ _ _ _ _ _ _]
            frame "Idle" {
            }
            frame "IntervalLineInt" {
            }
            frame "Ram Record" {
              w391 = 1 items=["Snap", "Sequence"] ("Capture mode")
              w414 = 0 items=["Snap", "Sequence"] ("Capture mode")
              n149 = call "tm_stopcapture.vi"("error in (no error)"=w417, "Handle in"=w401) -> ("error out"=w418:errorcluster, "Handle out"=w419:u32)  [unwired: 8 in]
              n150 = call "tm_unpreparecapture.vi"("error in (no error)"=w418, "Handle in"=w419) -> ("error out"=w416:errorcluster, "Handle out"=w415:u32)  [unwired: 8 in]
              n151 = call "tm_preparecapture.vi"("error in (no error)"=w416, "Frames"="Frames", "Capture mode"=w414, "Handle in"=w415) -> ("error out"=w412:errorcluster, "Buffer Info"=w392:T5, "Handle out"=w413:u32)  [unwired: 4 in, 1 out]
              n152 = call "tm_startcapture_b.vi"("error in (no error)"=w412, "Handle in"=w413) -> ("error out"=w393:errorcluster, "Handle out"=w411:u32)  [unwired: 8 in]
              n153 = Bundle("Mode"=ModeEnum."runWaves", "Microscope Settings"=w395) -> (w394:cluster{"Mode":T7, "Microscope Settings":T1})  [unwired: 1 in]
              n154 = Enqueue Element(queue=w397, element=w394, error in (no error)=w393) -> ()  [unwired: 1 in, 3 out]
              n155 = for {
                N: "Frames" -> [_]
                tunnel: w393 -> [w435]
                tunnel: w411 -> [w434]
                tunnel: w410 -> [w428]
                tunnel: [w426] -> w406
                tunnel: [w425] -> w405
                tunnel: w392 -> [w424]
                n156 = call "tm_waitnextframe.vi"("error in (no error)"=w435, "Handle in"=w434) -> ("error out"=w433:errorcluster, "Handle out"=w432:u32)  [unwired: 6 in, 2 out]
                n157 = call "tm_getframe_a.vi"("error in (no error)"=w433, "Buffer Info"=w424, "Handle in"=w432) -> ("error out"=w426:errorcluster, "Data 16"=w431:u16[][], "Handle out"=w425:u32)  [unwired: 4 in, 2 out]
                n158 = Bundle By Name(cluster=T10 {"State"=enum."Start Sequence", "Stack Number"=0, "Image"=[], "Stacks"=0} ("element"), "State"=Stack_Track."Save Image", "Stack Number"=0, "Image"=w431, "Stacks"=1) -> (w427:T10)
                n159 = Enqueue Element(queue=w428, element=w427) -> ()  [unwired: 2 in, 3 out]
              }
              n160 = call "tm_stopcapture.vi"("error in (no error)"=w406, "Handle in"=w405) -> ("error out"=w407:errorcluster, "Handle out"=w404:u32)  [unwired: 8 in]
              n161 = call "tm_unpreparecapture.vi"("error in (no error)"=w407, "Handle in"=w404) -> ("error out"=w408:errorcluster, "Handle out"=w403:u32)  [unwired: 8 in]
              n162 = call "tm_preparecapture.vi"("error in (no error)"=w408, "Capture mode"=w391, "Handle in"=w403) -> ("error out"=w409:errorcluster, "Buffer Info"=w390:T5, "Handle out"=w402:u32)  [unwired: 5 in, 1 out]
              n163 = call "tm_startcapture_b.vi"("error in (no error)"=w409, "Handle in"=w402) -> ("error out"=w399:errorcluster, "Handle out"=w400:u32)  [unwired: 8 in]
            }
            frame "HardDisk Record" {
            }
            frame "Disengage Update" {
            }
            frame "Update", Default {
              w447 = u32 2049184 items=["SENSOR MODE"=4212128, "CCD MODE"=4212384, "READOUT MODE"=4211872, "ACTIVE VIEW INDEX"=4343136, "BITS PER CHANNEL"=4342976, "IMAGE PIXEL TYPE"=4343296, "BINNING"=4215968, "EXPOSURE TIME"=2049184, "CONTRAST GAIN"=3163312, "CONTRAST OFFSET"=3163328, "LIGHT MODE"=2114720, "SENSITIVITY"=2114992, "PHOTON IMAGING MODE"=2115200, "HIGH DYNAMIC RANGE MODE"=3163360, "WHITE BALANCE"=3163568, "TEMPERATURE"=2115232, "TEMPERATURE TARGET"=2115264, "SENSOR COOLER FAN"=2115296, "LINEBUNDLE HEIGHT"=4212192, "MECHANICAL SHUTTER"=2115488, "BACK FOCUS POSITION"=8422304, "TRIGGER CONNECTOR"=1066432, "TRIGGER SOURCE"=1066144, "OUTPUT TRIGGER SOURCE"=1852576, "TRIGGER GLOBAL EXPOSURE"=2049680, "FIRST TRIGGER BEHAVIOR"=2049696, "CHANNEL SYNC"=1852352, "READOUT DIRECTION"=4211904, "PRE HSYNC COUNT"=1852704, "INTERNAL LINE SPEED"=4226000, "INTERNAL LINE INTERVAL"=4226016] ("Parameter")
              n164 = Unbundle By Name(w450) -> ("Exposure/ms"=w449:dbl)  [unwired: 1 out]
              n165 = Divide(x=w449, y=1000.0) -> (x/y=w446:dbl)
              n166 = call "tm_setparameter_a.vi"("Value in"=w446, "Parameter"=w447, "Handle in"=w452) -> ("Handle out"=w451:u32)  [unwired: 7 in, 1 out]
            }
            frame "ROI" {
            }
            frame "Binning" {
            }
            frame "Scan Mode" {
            }
            frame "Trigger Mode" {
            }
            frame "Readout Mode" {
              w483 = 1 items=["Snap", "Sequence"] ("Capture mode")
              w489 = u32 4194832  # Sensor Mode
              w492 = u32 2031888  # Exposure time
              n167 = Unbundle By Name(w502) -> ("Exposure/ms"=w501:dbl, "Slit.Slit Width /%"=w497:dbl, "Slit.Scanning Mode"=w487:dbl)
              n168 = call "tm_stopcapture.vi"("error in (no error)"=w503, "Handle in"=w505) -> ("error out"=w506:errorcluster, "Handle out"=w504:u32)  [unwired: 8 in]
              n169 = Divide(x=w501, y=1000.0) -> (x/y=w499:dbl)
              n170 = Multiply(x=w497, y=2048 ("input variable")) -> (x*y=w496:dbl)
              n171 = call "tm_unpreparecapture.vi"("error in (no error)"=w506, "Handle in"=w504) -> ("error out"=w484:errorcluster, "Handle out"=w488:u32)  [unwired: 8 in]
              n172 = call "tm_setpropertyvalue.vi"("error in (no error)"=w484, "Value in"=w487, "Property ID"=w489, "Handle in"=w488) -> ("error out"=w485:errorcluster, "Handle out"=w486:u32)  [unwired: 6 in]
              n173 = Divide(x=w496, y=100.0) -> (x/y=w494:dbl)
              n174 = case shown="1, Default" w487 {
                tunnel: [w511 w512] -> w493
                tunnel: w499 -> [w511 w520]
                tunnel: w494 -> [_ w519]
                tunnel: w486 -> [w510 w514]
                tunnel: [w510 w516] -> w491
                tunnel: [w509 w515] -> w490
                tunnel: w485 -> [w509 w513]
                frame 1, Default {
                }
                frame 12 {
                  w518 = u32 4208720  # Line Interval
                  n175 = formula code="slitExpos=frameInter*LW/(LinesToReadout\n+10+LW);\nlineInter = slitExpos / LW;"("frameInter"=w520, "LW"=w519, "LinesToReadout"=2048 ("input variable")) -> ("slitExpos"=w512:dbl, "lineInter"=w517:dbl)
                  n176 = call "tm_setpropertyvalue.vi"("error in (no error)"=w513, "Value in"=w517, "Property ID"=w518, "Handle in"=w514) -> ("error out"=w515:errorcluster, "Handle out"=w516:u32)  [unwired: 6 in]
                }
              }
              n177 = call "tm_setpropertyvalue.vi"("error in (no error)"=w490, "Value in"=w493, "Property ID"=w492, "Handle in"=w491) -> ("error out"=w478:errorcluster, "Handle out"=w480:u32)  [unwired: 6 in]
              n178 = call "tm_preparecapture.vi"("error in (no error)"=w478, "Capture mode"=w483, "Handle in"=w480) -> ("error out"=w482:errorcluster, "Handle out"=w481:u32)  [unwired: 5 in, 2 out]
              n179 = call "tm_startcapture_b.vi"("error in (no error)"=w482, "Handle in"=w481) -> ("error out"=w477:errorcluster, "Handle out"=w479:u32)  [unwired: 8 in]
            }
            frame "Readout Direction" {
            }
            frame "Preview" {
              n180 = call "tm_waitnextframe.vi"("error in (no error)"=w529, "Timeout"=500, "Handle in"=w535) -> ("error out"=w527:errorcluster, "Handle out"=w534:u32)  [unwired: 5 in, 2 out]
              n181 = case shown="No Error" w527 {
                selector: w527 -> [w538 w552]
                tunnel: w534 -> [w550 w551]
                tunnel: [w549 w551] -> w533
                tunnel: w531 -> [w548 _]
                tunnel: w530 -> [w547 _]
                tunnel: w529 -> [w542 _]
                tunnel: [w539 w552] -> w528
                frame No Error {
                  w544 = 0 ("Timeout")
                  n182 = call "tm_getframe_a.vi"("error in (no error)"=w538, "Buffer Info"=w548, "Handle in"=w550) -> ("error out"=w540:errorcluster, "Data 16"=w545:u16[][], "Handle out"=w549:u32)  [unwired: 4 in, 2 out]
                  n183 = Bundle("State"=Stack_Track."Display", "Timeout"=w544, "Data 16"=w545, "Timeout"=w544) -> (w543:T15)  [unwired: 1 in]
                  n184 = Enqueue Element(queue=w547, element=w543, error in (no error)=w542) -> (error out=w541:errorcluster)  [unwired: 1 in, 2 out]
                  n185 = Merge Errors(w540, w541) -> (w539:errorcluster)
                }
                frame Error {
                }
              }
            }
            frame "ROIWindow" {
            }
            frame "Trigger Source" {
              (unwired) u32 1066144 items=["SENSOR MODE"=4212128, "CCD MODE"=4212384, "READOUT MODE"=4211872, "ACTIVE VIEW INDEX"=4343136, "BITS PER CHANNEL"=4342976, "IMAGE PIXEL TYPE"=4343296, "BINNING"=4215968, "EXPOSURE TIME"=2049184, "CONTRAST GAIN"=3163312, "CONTRAST OFFSET"=3163328, "LIGHT MODE"=2114720, "SENSITIVITY"=2114992, "PHOTON IMAGING MODE"=2115200, "HIGH DYNAMIC RANGE MODE"=3163360, "WHITE BALANCE"=3163568, "TEMPERATURE"=2115232, "TEMPERATURE TARGET"=2115264, "SENSOR COOLER FAN"=2115296, "LINEBUNDLE HEIGHT"=4212192, "MECHANICAL SHUTTER"=2115488, "BACK FOCUS POSITION"=8422304, "TRIGGER CONNECTOR"=1066432, "TRIGGER SOURCE"=1066144, "OUTPUT TRIGGER SOURCE"=1852576, "TRIGGER GLOBAL EXPOSURE"=2049680, "FIRST TRIGGER BEHAVIOR"=2049696, "CHANNEL SYNC"=1852352, "READOUT DIRECTION"=4211904, "PRE HSYNC COUNT"=1852704, "INTERNAL LINE SPEED"=4226000, "INTERNAL LINE INTERVAL"=4226016] ("Parameter")
              w566 = 1 items=["Snap", "Sequence"] ("Capture mode")
              n186 = Unbundle By Name(w560) -> ("Mode"=w559:enum16{"X", "XY", "XYZ", "XYZT", "XYZC"})
              n187 = call "tm_stopcapture.vi"("error in (no error)"=w567, "Handle in"=w570) -> ("error out"=w574:errorcluster, "Handle out"=w575:u32)  [unwired: 8 in]
              n188 = call "tm_unpreparecapture.vi"("error in (no error)"=w574, "Handle in"=w575) -> ("error out"=w562:errorcluster, "Handle out"=w565:u32)  [unwired: 8 in]
              n189 = case shown="\"XYZT\"" w559 {
                tunnel: [T9 {"Mode"=2, "Polarity"=2, "Times"=2, "Delay"=0.0} ("Parameters") T9 {"Mode"=2, "Polarity"=2, "Times"=2, "Delay"=0.0} ("Parameters") T9 {"Mode"=2, "Polarity"=2, "Times"=2, "Delay"=0.0} ("Parameters") T9 {"Mode"=1, "Polarity"=2, "Times"=2, "Delay"=0.0} ("Parameters") T9 {"Mode"=1, "Polarity"=2, "Times"=2, "Delay"=0.0} ("Parameters")] -> w563
                tunnel: [CameraControlTypeDef."Preview" ("Enum") CameraControlTypeDef."Idle" ("Enum") CameraControlTypeDef."Idle" ("Enum") CameraControlTypeDef."Idle" ("Enum") CameraControlTypeDef."Preview" ("Enum")] -> w558
                frame "XY", Default {
                }
                frame "XYZT" {
                }
                frame "XYZ" {
                }
                frame "XYZC" {
                }
                frame "X" {
                }
              }
              n190 = call <userlib>:"tm_setinputtrigger.vi"("error in (no error)"=w562, "Parameters"=w563, "Handle in"=w565) -> ("error out"=w561:errorcluster, "Handle out"=w564:u32)  [unwired: 7 in]
              n191 = call "tm_preparecapture.vi"("error in (no error)"=w561, "Capture mode"=w566, "Handle in"=w564) -> ("error out"=w573:errorcluster, "Buffer Info"=w571:T5, "Handle out"=w572:u32)  [unwired: 5 in, 1 out]
              n192 = call "tm_startcapture_b.vi"("error in (no error)"=w573, "Handle in"=w572) -> ("error out"=w568:errorcluster, "Handle out"=w569:u32)  [unwired: 8 in]
            }
          }
          n193 = local read "stop"() -> (w359:bool)
        }
        n194 = while "Tiff Consumer" {
          tunnel: [w310] -> w163
          tunnel: [w319] -> w160
          tunnel: w154 -> [w321]
          tunnel: w153 -> [w314]
          shift-right: [w312] -> _
          shift-left: _ -> [_]
          stop <- w323 stop-if-true
          # "Delay, maybe?\nCheck"
          n195 = Dequeue Element(queue=w321, timeout in ms (-1)=1) -> (queue out=w318:refnum<queue>, element=w320:T10, error out=w317:errorcluster)  [unwired: 1 in, 1 out]
          n196 = Unbundle By Name(w320) -> ("State"=w315:T11, "Image"=w316:u16[][])  [unwired: 1 out]
          n197 = case shown="\"Save Image\"" w315 {
            tunnel: [w329 w332 w334 w338 w341 w344 w347 w355] -> w319
            tunnel: w318 -> [w329 w332 w334 w338 w341 w344 w347 w355]
            tunnel: w316 -> [w325 _ _ _ _ _ _ w354]
            tunnel: w314 -> [w328 w330 w333 w336 w339 w342 w345 w352]
            tunnel: w317 -> [w327 w331 w335 w337 w340 w343 w346 w353]
            tunnel: [w326 w331 w335 w337 w340 w343 w346 w351] -> w311
            tunnel: [w324 w330 w333 w336 w339 w342 w345 w348] -> w312
            frame "Display" {
              n198 = call "IMAQ ArrayToImage"("Image Pixels (U16)"=w325, "error in (no error)"=w327, "Image"=w328) -> ("error out"=w326:errorcluster, "Image Out"=w324:T3)  [unwired: 7 in]
            }
            frame "Idle", Default {
            }
            frame "Start Sequence" {
            }
            frame "Read Disk" {
            }
            frame "STOP" {
            }
            frame "Collecting" {
            }
            frame "End" {
            }
            frame "Save Image" {
              n199 = call "4Digit File Incrementer.vi"("path"="Imaging Folder") -> ("appended path"=w349:path)  [unwired: 10 in]
              "appended path" <- w349
              n200 = call "IMAQ ArrayToImage"("Image Pixels (U16)"=w354, "error in (no error)"=w353, "Image"=w352) -> ("error out"=w351:errorcluster, "Image Out"=w348:T3)  [unwired: 7 in]
              n201 = local write "Imaging Folder"(w349) -> ()
              n202 = call-poly "IMAQ Write File 2"("File Path"=w349, "Image"=w348) -> ()  [unwired: 8 in, 2 out]
            }
          }
          "Image" <- w312
          n203 = call "IMAQ Histograph"("error in (no error)"=w311, "Image"=w312) -> ("error out"=w310:errorcluster, "Histogram Graph"=→"Histogram":T4)  [unwired: 6 in, 2 out]
          n204 = local read "stop"() -> (w323:bool)
        }
        n205 = Merge Errors(w162, w163, w143) -> (w164:errorcluster)
      }
      frame "deinit" {
        n206 = call <vilib>:"DAQmx Stop Task.vi"("task/channels in"=w692) -> ("task out"=w693:refnum<k21>)  [unwired: 13 in, 1 out]
        n207 = call <vilib>:"DAQmx Stop Task.vi"("task/channels in"=w694) -> ("task out"=w695:refnum<k21>)  [unwired: 13 in, 1 out]
        n208 = call <vilib>:"DAQmx Clear Task.vi"("task in"=w693) -> ("error out"=w689:errorcluster)  [unwired: 14 in]
        n209 = call "tm_stopcapture.vi"("error in (no error)"=w704, "Handle in"=w700) -> ("error out"=w707:errorcluster, "Handle out"=w706:u32)  [unwired: 8 in]
        n210 = call <vilib>:"DAQmx Clear Task.vi"("task in"=w695) -> ("error out"=w690:errorcluster)  [unwired: 14 in]
        n211 = call "tm_unpreparecapture.vi"("error in (no error)"=w707, "Handle in"=w706) -> ("error out"=w708:errorcluster, "Handle out"=w705:u32)  [unwired: 8 in]
        n212 = call "tm_closecamera.vi"("error in (no error)"=w708, "Handle in"=w705) -> ("error out"=w709:errorcluster)  [unwired: 9 in]
        n213 = Flush Queue(queue=w682) -> (queue out=w688:refnum<queue>)  [unwired: 1 in, 2 out]
        n214 = call "tm_deinitialize.vi"("error in (no error)"=w709) -> ("error out"=w685:errorcluster)  [unwired: 10 in]
        n215 = Release Queue(queue=w683, error in (no error)=w685) -> (error out=w702:errorcluster)  [unwired: 1 in, 2 out]
        n216 = Release Queue(queue=w688) -> (error out=w691:errorcluster)  [unwired: 2 in, 2 out]
        n217 = Flush Queue(queue=w687, error in (no error)=w685) -> (queue out=w686:refnum<queue>, error out=w684:errorcluster)  [unwired: 1 out]
        n218 = Release Queue(queue=w686, error in (no error)=w684) -> (error out=w701:errorcluster)  [unwired: 1 in, 2 out]
        n219 = Merge Errors(w702, w701, w691, w690, w689) -> (w703:errorcluster)
      }
    }
    n220 = Or(x="stop", y=w18) -> (x .or. y?=w19:bool)
  }
  "error IO" <- w6
  n221 = disable-structure shown="Enabled" {
    frame Disabled {
      # "Parallise decode buffer"
      n222 = call "tm_startcapture_b.vi"() -> ()  [unwired: 10 in, 2 out]
      n223 = call "tm_waitnextframe.vi"() -> ()  [unwired: 8 in, 4 out]
      n224 = call "tm_getframe_a.vi"() -> ()  [unwired: 7 in, 5 out]
    }
    frame Enabled {
    }
  }
